vi "ReadErrorsH.vi"() -> ()   [LabVIEW 2010]
panel:
  in  "EDS_Errors":u32(ring) items=["OK"=0, "UNIMPLEMENTED"=1, "INTERNAL ERROR"=2, "MEM ALLOC FAILED"=3, "MEM FREE FAILED"=4, "OPERATION CANCELLED"=5, "INCOMPATIBLE VERSION"=6, "NOT SUPPORTED"=7, "UNEXPECTED EXCEPTION"=8, "PROTECTION VIOLATION"=9, "MISSING SUBCOMPONENT"=10, "SELECTION UNAVAILABLE"=11, "FILE IO ERROR"=32, "FILE TOO MANY OPEN"=33, "FILE NOT FOUND"=34, "FILE OPEN ERROR"=35, "FILE CLOSE ERROR"=36, "FILE SEEK ERROR"=37, "FILE TELL ERROR"=38, "FILE READ ERROR"=39, "FILE WRITE ERROR"=40, "FILE PERMISSION ERROR"=41, "FILE DISK FULL ERROR"=42, "FILE ALREADY EXISTS"=43, "FILE FORMAT UNRECOGNIZED"=44, "FILE DATA CORRUPT"=45, "FILE NAMING NA"=46, "DIR NOT FOUND"=64, "DIR IO ERROR"=65, "DIR ENTRY NOT FOUND"=66, "DIR ENTRY EXISTS"=67, "DIR NOT EMPTY"=68, "PROPERTIES UNAVAILABLE"=80, "PROPERTIES MISMATCH"=81, "PROPERTIES NOT LOADED"=83, "INVALID PARAMETER"=96, "INVALID HANDLE"=97, "INVALID POINTER"=98, "INVALID INDEX"=99, "INVALID LENGTH"=100, "INVALID FN POINTER"=101, "INVALID SORT FN"=102, "DEVICE NOT FOUND"=128, "DEVICE BUSY"=129, "DEVICE INVALID"=130, "DEVICE EMERGENCY"=131, "DEVICE MEMORY FULL"=132, "DEVICE INTERNAL ERROR"=133, "DEVICE INVALID PARAMETER"=134, "DEVICE NO DISK"=135, "DEVICE DISK ERROR"=136, "DEVICE CF GATE CHANGED"=137, "DEVICE DIAL CHANGED"=138, "DEVICE NOT INSTALLED"=139, "DEVICE STAY AWAKE"=140, "DEVICE NOT RELEASED"=141, "STREAM IO ERROR"=160, "STREAM NOT OPEN"=161, "STREAM ALREADY OPEN"=162, "STREAM OPEN ERROR"=163, "STREAM CLOSE ERROR"=164, "STREAM SEEK ERROR"=165, "STREAM TELL ERROR"=166, "STREAM READ ERROR"=167, "STREAM WRITE ERROR"=168, "STREAM PERMISSION ERROR"=169, "STREAM COULDNT BEGIN THREAD"=170, "STREAM BAD OPTIONS"=171, "STREAM END OF STREAM"=172, "COMM PORT IS IN USE"=192, "COMM DISCONNECTED"=193, "COMM DEVICE INCOMPATIBLE"=194, "COMM BUFFER FULL"=195, "COMM USB BUS ERR"=196, "USB DEVICE LOCK ERROR"=208, "USB DEVICE UNLOCK ERROR"=209, "STI UNKNOWN ERROR"=224, "STI INTERNAL ERROR"=225, "STI DEVICE CREATE ERROR"=226, "STI DEVICE RELEASE ERROR"=227, "DEVICE NOT LAUNCHED"=228, "ENUM NA"=240, "INVALID FN CALL"=241, "HANDLE NOT FOUND"=242, "INVALID ID"=243, "WAIT TIMEOUT ERROR"=244, "SESSION NOT OPEN"=8195, "INVALID TRANSACTIONID"=8196, "INCOMPLETE TRANSFER"=8199, "INVALID STRAGEID"=8200, "DEVICEPROP NOT SUPPORTED"=8202, "INVALID OBJECTFORMATCODE"=8203, "SELF TEST FAILED"=8209, "PARTIAL DELETION"=8210, "SPECIFICATION BY FORMAT UNSUPPORTED"=8212, "NO VALID OBJECTINFO"=8213, "INVALID CODE FORMAT"=8214, "UNKNOWN VENDOR CODE"=8215, "CAPTURE ALREADY TERMINATED"=8216, "INVALID PARENTOBJECT"=8218, "INVALID DEVICEPROP FORMAT"=8219, "INVALID DEVICEPROP VALUE"=8220, "SESSION ALREADY OPEN"=8222, "TRANSACTION CANCELLED"=8223, "SPECIFICATION OF DESTINATION UNSUPPORTED"=8224, "UNKNOWN COMMAND"=40961, "OPERATION REFUSED"=40965, "LENS COVER CLOSE"=40966, "LOW BATTERY"=41217, "OBJECT NOTREADY"=41218, "TAKE PICTURE AF NG"=36097, "TAKE PICTURE RESERVED"=36098, "TAKE PICTURE MIRROR UP NG"=36099, "TAKE PICTURE SENSOR CLEANING NG"=36100, "TAKE PICTURE SILENCE NG"=36101, "TAKE PICTURE NO CARD NG"=36102, "TAKE PICTURE CARD NG"=36103, "TAKE PICTURE CARD PROTECT NG"=36104, "TAKE PICTURE MOVIE CROP NG"=36105, "TAKE PICTURE STROBO CHARGE NG"=36106, "LAST GENERIC ERROR PLUS ONE"=245]
  # "Copy-paste this control as type definition\nor \"customize\" it to save it in the library\nas type def"
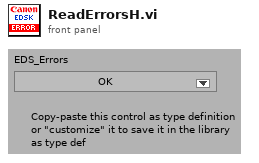
[diagram p1: front panel]
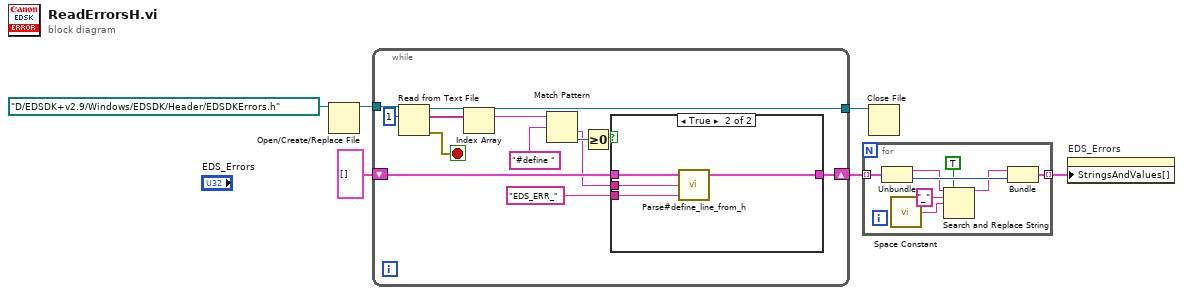
[diagram p0: block diagram]
diagram:
  n1 = Open/Create/Replace File(file path (use dialog)=path "D:/EDSDK+v2.9/Windows/EDSDK/Header/EDSDKErrors.h") -> (refnum out=w5:refnum<file>)  [unwired: 5 in, 2 out]
  n2 = while {
    tunnel: w5 -> [w19]
    tunnel: [w8] -> w4
    shift-right: [w13] -> w2
    shift-left: cluster{string, i32}[] [] -> [w14]
    stop <- w17 stop-if-true
    n3 = Read from Text File(file (use dialog)=w19, count=1) -> (refnum out=w8:refnum<file>, text=w10:string[], error out=w17:errorcluster)  [unwired: 2 in, 1 out]
    n4 = Index Array(array=w10) -> (element=w9:string)  [unwired: 1 in]
    n5 = Match Pattern(string=w9, regular expression="#define ") -> (after substring=w12:string, offset past match=w16:i32)  [unwired: 1 in, 2 out]
    n6 = Greater Or Equal To 0?(x=w16) -> (x >= 0?=w15:bool)
    n7 = case shown="True" w15 {
      tunnel: w14 -> [w20 w24]
      tunnel: [w20 w23] -> w13
      tunnel: w12 -> [_ w22]
      tunnel: "EDS_ERR_" ("regular expression") -> [_ w21]
      frame False {
      }
      frame True {
        n8 = call "Parse#define_line_from_h.vi"("define prefix"=w21, "define line"=w22, "define-values in"=w24) -> ("define-values out"=w23:cluster{string, u32}[])  [unwired: 2 in]
      }
    }
  }
  n9 = for {
    tunnel: w2 -> [w32] mode=indexing
    tunnel: [w30] -> w1 mode=indexing
    n10 = Unbundle(w32) -> (w29:string, w31:u32)
    n11 = call <vilib>:"Space Constant.vi"() -> ("String"=w27:string)
    n12 = Search and Replace String(replace all?=TRUE ("replace all? (F)"), input string=w29, search string="_", replace string=w27) -> (result string=w26:string)  [unwired: 4 in, 3 out]
    n13 = Bundle("result string"=w26, w31) -> (w30:cluster{"result string":string, u32})  [unwired: 1 in]
  }
  n14 = Close File(refnum=w4) -> ()  [unwired: 1 in, 2 out]
  n15 = property on="EDS_Errors" class="Ring (strict)"("StringsAndValues[]"=w1) -> ()  [unwired: 2 in, 2 out]
